vi "PH_Cont-601k_PowerUnit.scr Configure.vi"(0 "VI in":refnum<vi>, 5 "error in (no error)":errorcluster) -> (14 "VI out":refnum<vi>, 19 "error out":errorcluster)   [LabVIEW 2014, in "PH_Cont-601k_PowerUnit.lvlib"]
uses:
  PH_Cont-601k_PowerUnit.lvlib
  PH_Devices/PH_Cont-601k_PSU/PH_Cont-601k_PSU.Mode.ctl
  PH_Basics/PH_PowerUnit_BaseClass/PH_PowerUnit_BaseClass.SM States.ctl
  PH_Devices/PH_Cont-601k_PSU/PH_Cont-601k_PSU.lvlib
  PH_Basics/PH_PowerUnit_BaseClass/PH_PowerUnit_BaseClass.lvlib
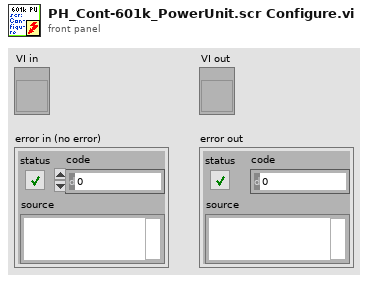
[diagram p1: front panel]
types:
  T1 = typedef "PH_PowerUnit_BaseClass.lvlib/PH_PowerUnit_BaseClass.SM States.ctl" = enum16{".", "Stand by", "Switch PU on", "Configure", "Set Default Voltage", "Set STANDBY", "Set READY", "Wait for Shot Cmd", "Open Dump Rods", "Open Ross Relais", "Close Ross Relais", "Switch PSU on", "Switch PSU off", "Charge", "Switch GD Channel on", "Close Dump Rods", "Rods-TO", "RR-TO", "PSU-TO", "Trigger-TO"}
  T2 = typedef "PH_Cont-601k_PSU.lvlib/PH_Cont-601k_PSU.Mode.ctl" = enum32{"STOP", "STANDBY", "READY", "EMISSION", "ERROR"}
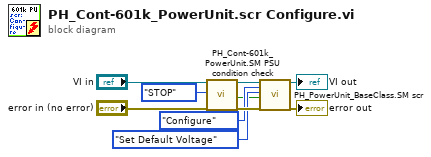
[diagram p0: block diagram]
diagram:
  n1 = call "PH_Cont-601k_PowerUnit.SM PSU condition check.vi"("VI in"="VI in", "Wanted Device Mode (READY)"=PH_Cont-601k_PSU.Mode."STOP" ("y"), "error in (no error)"="error in (no error)") -> ("VI out"=w9:refnum<vi>, "Condition fullfilled"=w2:bool, "error out"=w10:errorcluster)  [unwired: 14 in]
  n2 = call "PH_PowerUnit_BaseClass.SM scr.vi"("VI in"=w9, "Current SM State (condition)"=PH_PowerUnit_BaseClass.SM_States."Configure", "Wanted SM State"=PH_PowerUnit_BaseClass.SM_States."Set Default Voltage", "Further change condition"=w2, "error in (no error)"=w10) -> ("VI out"=→"VI out":refnum<vi>, "error out"=→"error out":errorcluster)  [unwired: 13 in]
